vi "Enum String to Symbol.vi"(10 "Symbol String In":string(combo)="PWM Out") -> (2 "Symbol Enum Out":T1)   [LabVIEW 2013]
uses:
  enum_Symbols.ctl
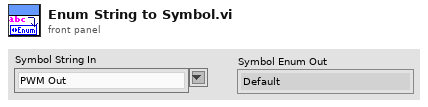
[diagram p1: front panel]
types:
  T1 = typedef "enum_Symbols.ctl" = enum16{"Default", "Analog Input", "Analog Output", "Digital Input", "Digital Output", "PWM Input", "PWM Output"}
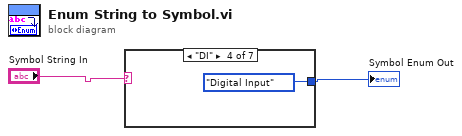
[diagram p0: block diagram]
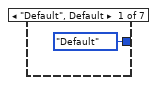
[diagram p2: hidden frame]
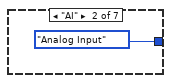
[diagram p3: hidden frame]
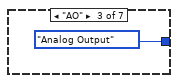
[diagram p4: hidden frame]
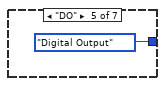
[diagram p5: hidden frame]
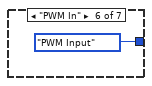
[diagram p6: hidden frame]
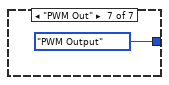
[diagram p7: hidden frame]
diagram:
  n1 = case shown="\"DI\"" "Symbol String In" {
    tunnel: [enum_Symbols."Default" ("Symbol Enum In") enum_Symbols."Analog Input" ("Symbol Enum In") enum_Symbols."Analog Output" ("Symbol Enum In") enum_Symbols."Digital Input" ("Symbol Enum In") enum_Symbols."Digital Output" ("Symbol Enum In") enum_Symbols."PWM Input" ("Symbol Enum In") enum_Symbols."PWM Output" ("Symbol Enum In")] -> w2
    frame "Default", Default {
    }
    frame "AI" {
    }
    frame "AO" {
    }
    frame "DI" {
    }
    frame "DO" {
    }
    frame "PWM In" {
    }
    frame "PWM Out" {
    }
  }
  "Symbol Enum Out" <- w2
